vi "Calibration LastCal (Read).vi"(6 "ISOBUS address":T2=-1 caption="ISOBUS address (-1)", 8 "error in":errorcluster, 11 "Mercury Reference In":T3) -> (0 "error out":errorcluster, 2 "Time of Last Calibration (ms)":string, 3 "Mercury Reference Out":T3, 4 "Valid?":T1)   [LabVIEW 2019, in "Mercury iXX.lvlib" / "Temperature.lvlib"]
doc: "Read the current calibration file for the selected temperature device."
uses:
  Temperature.lvlib
  Controls/Mercury Reference.ctl
  Controls/Comms Transport Layer.ctl
  Private/Controls/Query Dynamic Reference.ctl
  Controls/ISOBus Address.ctl
  Controls/Is Valid LED.ctl
  Private/Controls/Command Verbs.ctl
  Mercury iXX.lvlib
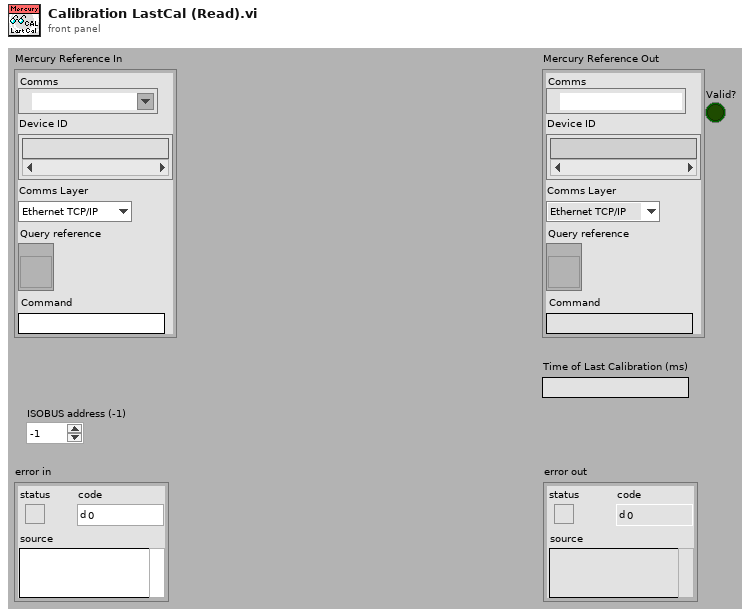
[diagram p1: front panel]
types:
  T1 = typedef "Mercury iXX.lvlib/Is Valid LED.ctl" = bool
  T2 = typedef "Mercury iXX.lvlib/ISOBus Address.ctl" = i32
  T3 = typedef "Mercury iXX.lvlib/Mercury Reference.ctl" = cluster{"Comms":refnum<visa-resource-name>, "Device ID":string[], "Comms Layer":T4, "Command":string, "Query reference":T5}
  T4 = typedef "Mercury iXX.lvlib/Comms Transport Layer.ctl" = enum16{"Ethernet TCP/IP", "USB", "ISOBus - RS-232", "GPIB"}
  T5 = typedef "Mercury iXX.lvlib/Query Dynamic Reference.ctl" = refnum<vi>
  T6 = typedef "Mercury iXX.lvlib/Command Verbs.ctl" = string
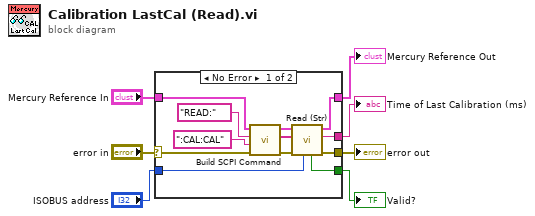
[diagram p0: block diagram]
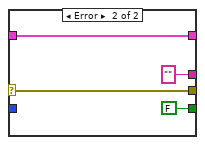
[diagram p2: hidden frame]
diagram:
  n1 = case shown="No Error" "error in" {
    selector: "error in" -> [w10 w23]
    tunnel: "Mercury Reference In" -> [w16 w22]
    tunnel: [w15 w22] -> w6
    tunnel: "ISOBUS address" -> [w14 _]
    tunnel: [w13 T1 FALSE ("Valid?")] -> w4
    tunnel: [w12 w23] -> w3
    tunnel: [w11 "" ("Response")] -> w2
    frame No Error {
      n2 = call "Build SCPI Command.vi"("error in"=w10, "Noun(s)"=":CAL:CAL" ("Command"), "Verb"=T6 "READ:", "Mercury Reference In"=w16) -> ("error out"=w17:errorcluster, "SCPI Message(s)"=w19:string[], "Mercury Reference Out"=w18:T3)  [unwired: 5 out]
      n3 = call "Read (Str).vi"("ISOBUS address"=w14, "error in"=w17, "SCPI Message(s)"=w19, "Mercury Reference In"=w18) -> ("error out"=w12:errorcluster, "Response"=w11:string, "Mercury Reference Out"=w15:T3, "Valid?"=w13:T1)  [unwired: 4 out]
    }
    frame Error {
    }
  }
  "Mercury Reference Out" <- w6
  "error out" <- w3
  "Time of Last Calibration (ms)" <- w2
  "Valid?" <- w4
